vi "Test Settings API.vi"() -> ()   [LabVIEW 2020]
doc: "Settings API Tester."
uses:
  Acquisition/cluster analogico.ctl
  Acquisition/cluster digital.ctl
  Settings.lvlib
  Acquisition/CONTROLS.lvlib
panel:
  out "NAME":string
  out "ACTIVIDADES":string[][](table)
  in  "Erase all":bool
  in  "ANALOGICO/DIGITAL":bool
  in  "Adquisicion tiempo":i32
  in  "DAQ BOARD":tag
  in  "DIGITAL":T1={"Puertos Digital"=[], "Lineas Digital"=[], "Frecuencia Muestreo"=1000, "Puerto/Linea"=FALSE}
  in  "ANALOGICO":T2={"ANALOGICO CANALES"=[], "Numero de muestras"=1000, "Frecuencia de muestreo"=1000}
  in  "ADD TASK":bool
  in  "Show Block Diagram":bool
  in  "Stop Module":bool
  in  "Start Module":bool
  in  "Hide Module Panel":bool
  in  "Show Module Panel":bool
  out "Status":string
  out "Module Running?":bool
  # "This VI tests the API for the Module."
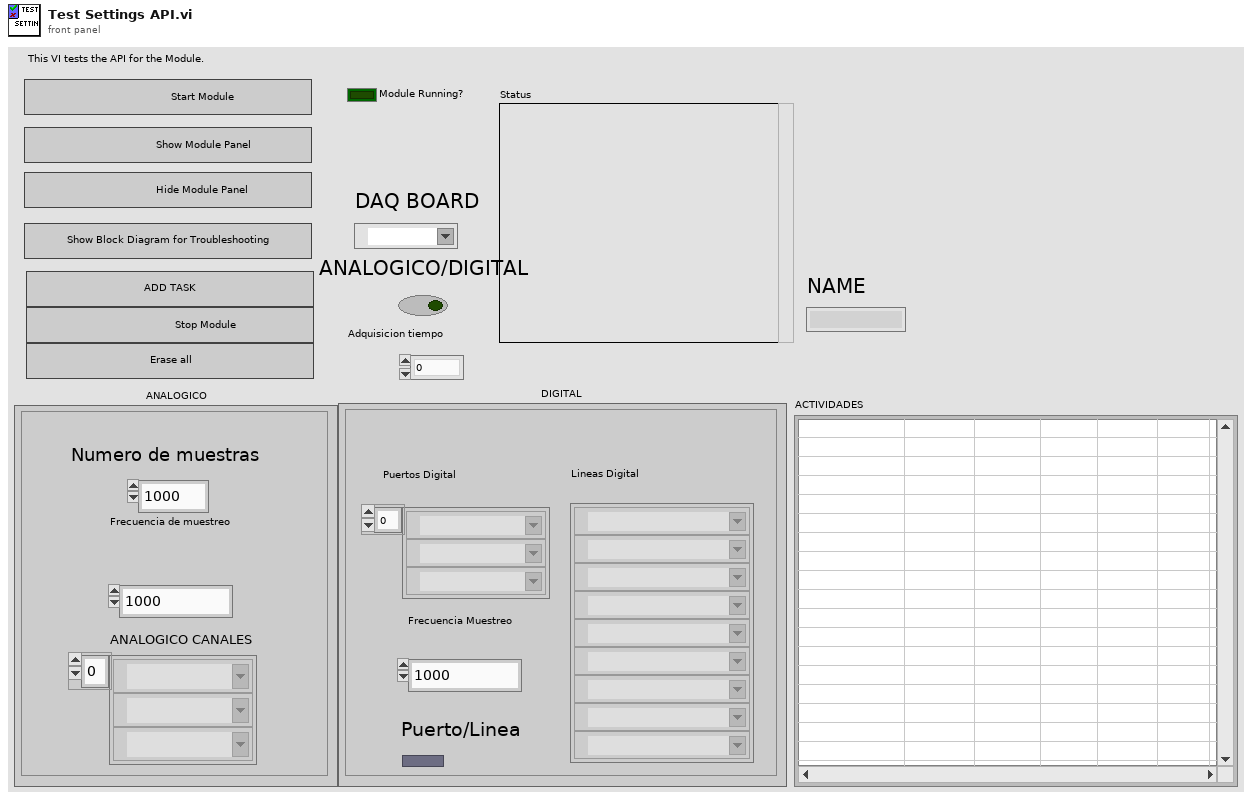
[diagram p1: front panel]
types:
  T1 = typedef "Acquisition.lvlib/CONTROLS.lvlib/cluster digital.ctl" = cluster{"Puertos Digital":tag[], "Lineas Digital":tag[], "Frecuencia Muestreo":u32, "Puerto/Linea":bool}
  T2 = typedef "Acquisition.lvlib/CONTROLS.lvlib/cluster analogico.ctl" = cluster{"ANALOGICO CANALES":tag[], "Numero de muestras":u32, "Frecuencia de muestreo":u32}
  T3 = typedef "Settings.lvlib/Broadcast Events--cluster.ctl" = cluster{"Module Did Init":refnum<user-event>, "Status Updated":refnum<user-event>, "Error Reported":refnum<user-event>, "Module Did Stop":refnum<user-event>, "Update Module Execution Status":refnum<user-event>, "Task to do":refnum<user-event>, "Nombre task":refnum<user-event>}
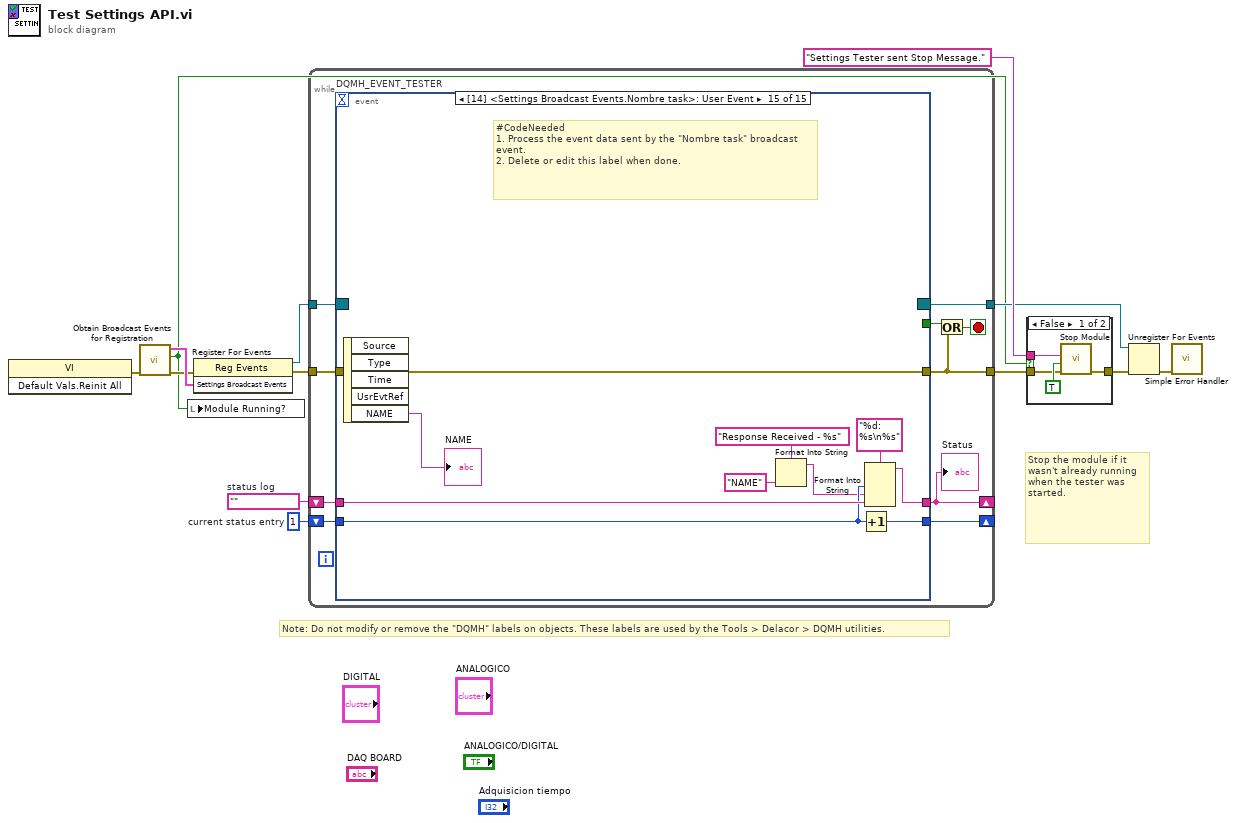
[diagram p0: block diagram]
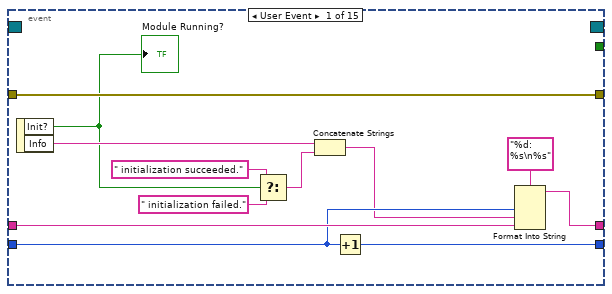
[diagram p3: hidden frame]
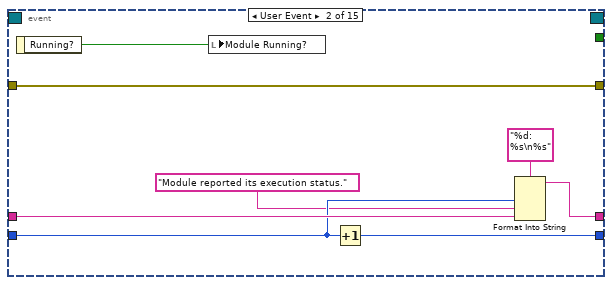
[diagram p4: hidden frame]
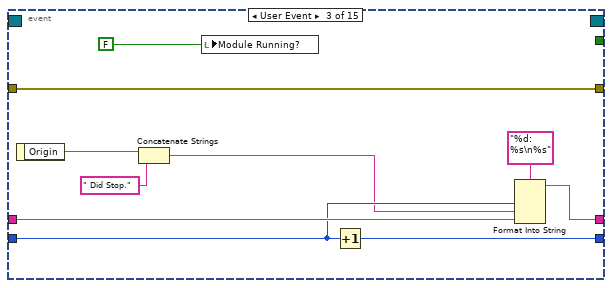
[diagram p5: hidden frame]
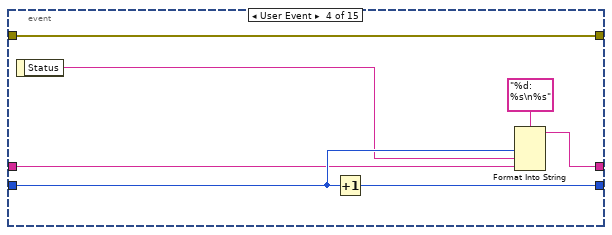
[diagram p6: hidden frame]
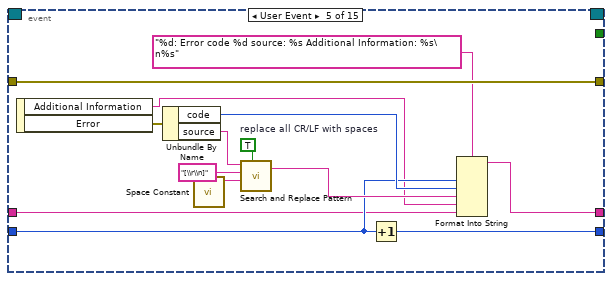
[diagram p7: hidden frame]
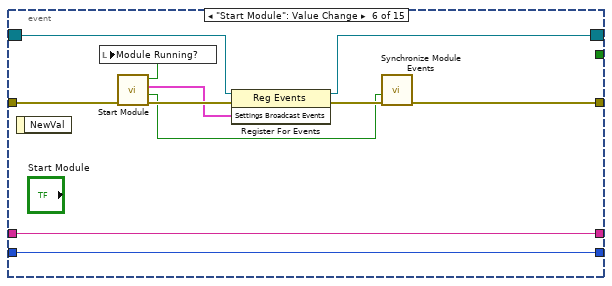
[diagram p8: hidden frame]
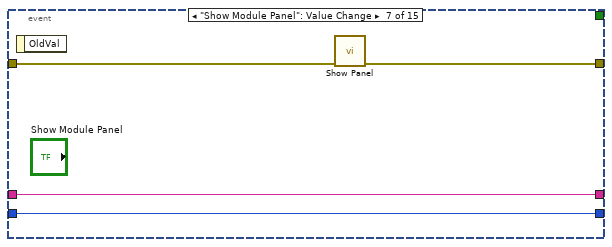
[diagram p9: hidden frame]
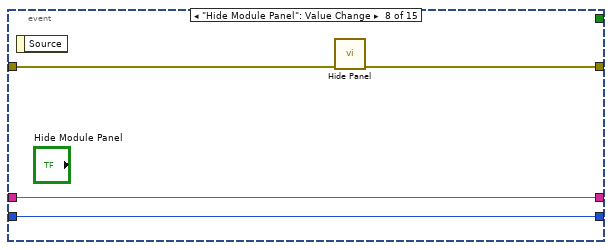
[diagram p10: hidden frame]
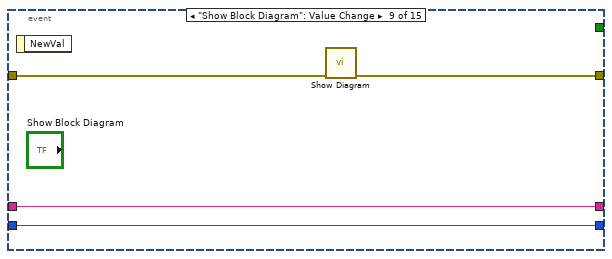
[diagram p11: hidden frame]
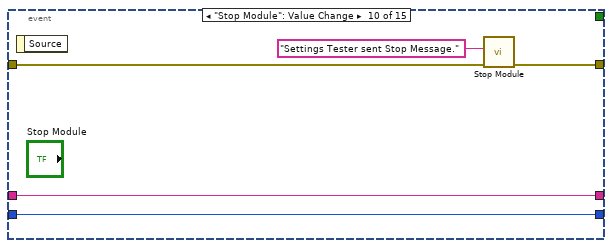
[diagram p12: hidden frame]
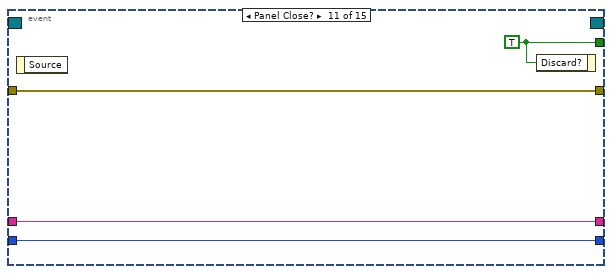
[diagram p13: hidden frame]
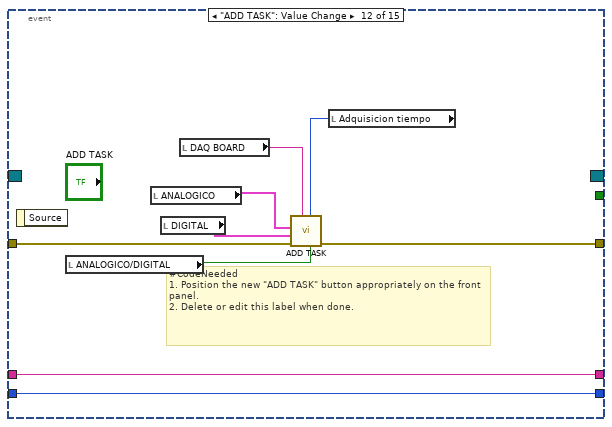
[diagram p14: hidden frame]
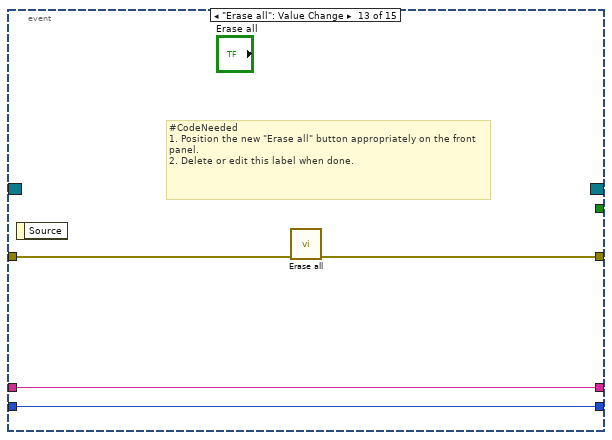
[diagram p15: hidden frame]
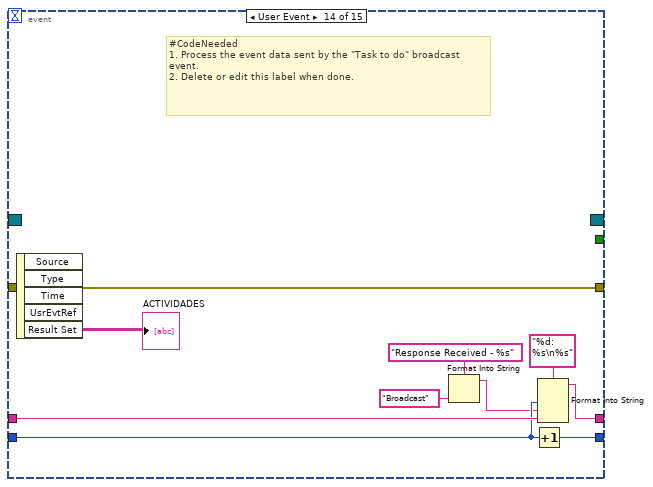
[diagram p16: hidden frame]
diagram:
  w10 = 1  # current status entry
  w11 = ""  # status log
  # "Stop the module if it wasn't already running when the tester was started."
  # "Note: Do not modify or remove the \"DQMH\" labels on objects. These labels are used by the Tools > Delacor > DQMH utilities."
  n1 = invoke class="VI" method="Default Vals.Reinit All"() -> (error out=w5:errorcluster)  [unwired: 3 in, 2 out]
  n2 = call "Obtain Broadcast Events for Registration.vi"("error in (no error)"=w5) -> ("error out"=w4:errorcluster, "Already running?"=w3:bool, "Settings Broadcast Events"=w8:T3)  [unwired: 8 in]
  n3 = local write "Module Running?"(w3) -> ()
  n4 = register-events(error in=w4, w8) -> (reference out=w7:refnum<event-registration>, error out=w9:errorcluster)  [unwired: 1 in]
  n5 = while {
    tunnel: w7 -> [w23]
    tunnel: [w14] -> w2
    shift-right: [w18] -> _
    shift-left: w11 -> [w20]
    shift-right: [w19] -> _
    shift-left: w10 -> [w21]
    tunnel: w9 -> [w16]
    tunnel: [w15] -> w6
    stop <- w17 stop-if-true
    n6 = event "DQMH_EVENT_TESTER" shown="[14] <Settings Broadcast Events.Nombre task>: User Event" {
      selector: w23 -> [_ _ _ _ _ w79 _ _ _ _ _ _ _ _ _]
      dyn-events: [_ _ _ _ _ w78 _ _ _ _ _ _ _ _ _] -> w15
      timeout: _ -> [_ _ _ _ _ _ _ _ _ _ _ _ _ _ _]
      tunnel: [_ _ _ _ _ _ _ _ _ _ w106 _ _ _ _] -> w22
      tunnel: [w35 w37 w44 w54 w74 w77 w89 w93 w94 w100 w103 w112 w116 w129 w139] -> w14
      tunnel: w21 -> [w32 w41 w51 w57 w64 w82 w87 w91 w95 w101 w104 w113 w117 w126 w136]
      tunnel: w20 -> [w33 w42 w52 w56 w62 w83 w88 w92 w96 w102 w105 w114 w118 w128 w138]
      tunnel: [w30 w39 w49 w58 w65 w83 w88 w92 w96 w102 w105 w114 w118 w127 w137] -> w18
      tunnel: [w31 w40 w50 w60 w63 w82 w87 w91 w95 w101 w104 w113 w117 w125 w135] -> w19
      tunnel: w16 -> [w35 w37 w44 w54 w74 w76 w86 w90 w97 w98 w103 w115 w119 w129 w139]
      event User Event {
        n7 = event-data() -> ("Init?"=w27:bool, "Info"=w29:string)  [unwired: 1 in]
        "Module Running?" <- w27
        n8 = Select(t=" initialization succeeded.", s=w27, f=" initialization failed.") -> (s? t:f=w24:string)
        n9 = Concatenate Strings(w29, w24) -> (w28:string)
        n10 = Increment(x=w32) -> (x+1=w31:i32)
        n11 = Format Into String(format string="%d: %s\n%s", w32, w28, w33) -> (resulting string=w30:string)  [unwired: 2 in, 1 out]
      }
      event User Event {
        n12 = event-data() -> ("Running?"=w36:bool)  [unwired: 1 in]
        n13 = local write "Module Running?"(w36) -> ()
        n14 = Increment(x=w41) -> (x+1=w40:i32)
        n15 = Format Into String(format string="%d: %s\n%s", w41, "Module reported its execution status.", w42) -> (resulting string=w39:string)  [unwired: 2 in, 1 out]
      }
      event User Event {
        n16 = event-data() -> ("Origin"=w48:string)  [unwired: 1 in]
        n17 = Concatenate Strings(w48, " Did Stop.") -> (w47:string)
        n18 = local write "Module Running?"(FALSE ("Module Did Init?")) -> ()
        n19 = Increment(x=w51) -> (x+1=w50:i32)
        n20 = Format Into String(format string="%d: %s\n%s", w51, w47, w52) -> (resulting string=w49:string)  [unwired: 2 in, 1 out]
      }
      event User Event {
        n21 = event-data() -> ("Status"=w55:string)  [unwired: 1 in]
        n22 = Increment(x=w57) -> (x+1=w60:i32)
        n23 = Format Into String(format string="%d: %s\n%s", w57, w55, w56) -> (resulting string=w58:string)  [unwired: 2 in, 1 out]
      }
      event User Event {
        w70 = TRUE  # replace all CR/LF with spaces
        n24 = event-data() -> ("Additional Information"=w61:string, "Error"=w66:errorcluster)  [unwired: 1 in]
        n25 = Unbundle By Name(w66) -> ("code"=w67:i32, "source"=w68:string)
        n26 = call <vilib>:"Space Constant.vi"() -> ("String"=w71:string)
        n27 = call <vilib>:"Search and Replace Pattern.vi"("string"=w68, "regular expression (\"\")"="[\\r\\n]" ("regular expression (\"\")"), "replace string (\"\")"=w71, "replace all? (F)"=w70) -> ("result string"=w69:string)  [unwired: 1 in, 1 out]
        n28 = Increment(x=w64) -> (x+1=w63:i32)
        n29 = Format Into String(format string="%d: Error code %d source: %s Additional Information: %s\n%s", w64, w67, w69, w61, w62) -> (resulting string=w65:string)  [unwired: 2 in, 1 out]
      }
      event "Start Module": Value Change {
        n30 = event-data() -> ()  [unwired: 1 in, 1 out]
        n31 = call "Start Module.vi"("error in (no error)"=w76) -> ("error out"=w84:errorcluster, "Wait for Event Sync?"=w81:bool, "Settings Broadcast Events"=w80:T3, "Module Was Already Running?"=w75:bool)  [unwired: 7 in]
        n32 = local write "Module Running?"(w75) -> ()
        n33 = register-events(reference=w79, error in=w84, w80) -> (reference out=w78:refnum<event-registration>, error out=w85:errorcluster)
        n34 = call "Synchronize Module Events.vi"("error in"=w85, "Wait for Event Sync?"=w81) -> ("error out"=w77:errorcluster)  [unwired: 9 in]
      }
      event "Show Module Panel": Value Change {
        n35 = event-data() -> ()  [unwired: 1 in, 1 out]
        n36 = call "Show Panel.vi"("error in (no error)"=w86) -> ("error out"=w89:errorcluster)  [unwired: 10 in]
      }
      event "Hide Module Panel": Value Change {
        n37 = event-data() -> ()  [unwired: 1 in, 1 out]
        n38 = call "Hide Panel.vi"("error in (no error)"=w90) -> ("error out"=w93:errorcluster)  [unwired: 10 in]
      }
      event "Show Block Diagram": Value Change {
        n39 = event-data() -> ()  [unwired: 1 in, 1 out]
        n40 = call "Show Diagram.vi"("error in (no error)"=w97) -> ("error out"=w94:errorcluster)  [unwired: 10 in]
      }
      event "Stop Module": Value Change {
        n41 = event-data() -> ()  [unwired: 1 in, 1 out]
        n42 = call "Stop Module.vi"("error in"=w98, "Origin"="Settings Tester sent Stop Message.") -> ("error out"=w100:errorcluster)  [unwired: 9 in]
      }
      event Panel Close? {
        w106 = TRUE ("Discard?")
        n43 = event-data() -> ()  [unwired: 1 in, 1 out]
        n44 = event-data("Discard?"=w106) -> ()  [unwired: 1 in, 1 out]
      }
      event "ADD TASK": Value Change {
        # "#CodeNeeded\n1. Position the new \"ADD TASK\" button appropriately on the front panel.\n2. Delete or edit this label when done."
        n45 = event-data() -> ()  [unwired: 1 in, 1 out]
        n46 = local read "ANALOGICO/DIGITAL"() -> (w107:bool)
        n47 = local read "ANALOGICO"() -> (w109:T2)
        n48 = local read "DIGITAL"() -> (w108:T1)
        n49 = local read "DAQ BOARD"() -> (w110:tag)
        n50 = local read "Adquisicion tiempo"() -> (w111:i32)
        n51 = call "ADD TASK.vi"("ANALOGICO/DIGITAL"=w107, "Adquisicion tiempo"=w111, "DAQ BOARD"=w110, "error in"=w115, "DIGITAL"=w108, "ANALOGICO"=w109) -> ("error out"=w112:errorcluster)  [unwired: 5 in]
      }
      event "Erase all": Value Change {
        # "#CodeNeeded\n1. Position the new \"Erase all\" button appropriately on the front panel.\n2. Delete or edit this label when done."
        n52 = event-data() -> ()  [unwired: 1 in, 1 out]
        n53 = call "Erase all.vi"("error in"=w119) -> ("error out"=w116:errorcluster)  [unwired: 10 in]
      }
      event User Event {
        # "#CodeNeeded\n1. Process the event data sent by the \"Task to do\" broadcast event.\n2. Delete or edit this label when done."
        n54 = event-data() -> ("Result Set"=→"ACTIVIDADES":string[][])  [unwired: 1 in, 4 out]
        n55 = Format Into String(format string="Response Received - %s", "Broadcast" ("input 1")) -> (resulting string=w122:string)  [unwired: 2 in, 1 out]
        n56 = Increment(x=w126) -> (x+1=w125:i32)
        n57 = Format Into String(format string="%d: %s\n%s", w126, w122, w128) -> (resulting string=w127:string)  [unwired: 2 in, 1 out]
      }
      event User Event {
        # "#CodeNeeded\n1. Process the event data sent by the \"Nombre task\" broadcast event.\n2. Delete or edit this label when done."
        n58 = event-data() -> ("NAME"=→"NAME":string)  [unwired: 1 in, 4 out]
        n59 = Format Into String(format string="Response Received - %s", "NAME" ("input 1")) -> (resulting string=w132:string)  [unwired: 2 in, 1 out]
        n60 = Increment(x=w136) -> (x+1=w135:i32)
        n61 = Format Into String(format string="%d: %s\n%s", w136, w132, w138) -> (resulting string=w137:string)  [unwired: 2 in, 1 out]
      }
    }
    "Status" <- w18
    n62 = Or(x=w22, y=w14) -> (x .or. y?=w17:bool)
  }
  n63 = case shown="False" w3 {
    tunnel: [w143 w144] -> w13
    tunnel: "Settings Tester sent Stop Message." ("Origin") -> [w142 _]
    tunnel: w2 -> [w140 w144]
    frame False {
      n64 = call "Stop Module.vi"("error in"=w140, "Wait for Module to Stop? (F)"=TRUE ("Wait for Module to stop?"), "Origin"=w142) -> ("error out"=w143:errorcluster)  [unwired: 8 in]
    }
    frame True {
    }
  }
  n65 = Unregister For Events(event registration refnum=w6, error in=w13) -> (error out=w1:errorcluster)
  n66 = call <vilib>:"Simple Error Handler.vi"("error in (no error)"=w1) -> ()  [unwired: 4 in, 5 out]
